vi "Toggle and Hold.vi"(7 "Reset? (F)":bool, 10 "Hold Time (ms)":u32, 11 "Trigger":bool) -> (3 "Toggled?":bool)   [LabVIEW 2019]
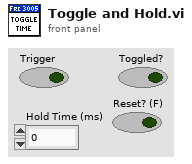
[diagram p1: front panel]
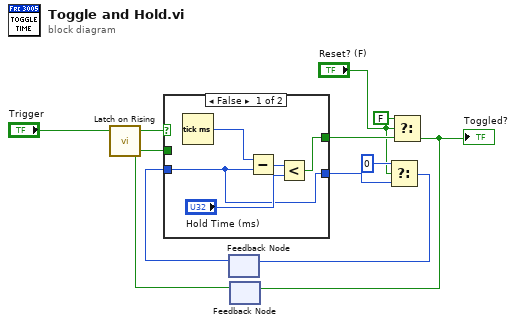
[diagram p0: block diagram]
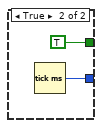
[diagram p2: hidden frame]
diagram:
  n1 = call <vilib>:"Latch on Rising.vi"("Boolean in"="Trigger") -> ("Boolean out"=w11:bool)  [unwired: 4 in]
  n2 = feedback #1() -> (w8:u32)  [unwired: 1 in]
  n3 = feedback #2() -> (w7:bool)  [unwired: 1 in]
  n4 = case shown="False" w11 {
    tunnel: [w12 w18] -> w9
    tunnel: w8 -> [w12 _]
    tunnel: [w13 TRUE] -> w5
    tunnel: w7 -> [_ _]
    frame False {
      n5 = Tick Count (ms)() -> (millisecond timer value=w16:u32)
      n6 = Subtract(x=w16, y=w12) -> (x-y=w15:u32)
      n7 = Less?(x=w15, y="Hold Time (ms)") -> (x < y?=w13:bool)
    }
    frame True {
      n8 = Tick Count (ms)() -> (millisecond timer value=w18:u32)
    }
  }
  n9 = Select(t=u32 0, s="Reset? (F)", f=w9) -> (s? t:f=w3:u32)
  n10 = feedback-in #1(w3) -> ()
  n11 = Select(t=FALSE, s="Reset? (F)", f=w5) -> (s? t:f=w6:bool)
  "Toggled?" <- w6
  n12 = feedback-in #2(w6) -> ()
